vi "example_01_compress.vi"() -> ()   [LabVIEW 2015, in "lv-bin-7zip.lvlib" / "v1.lvlib"]
uses:
  v1.lvlib
  <userlib>/antonio-alexander/lv-bin/lv-bin/public/api/v1/advanced/add_data_path_multiple.vi
  advanced/compress_exe.vi
  <userlib>/antonio-alexander/lv-bin/lv-bin/public/api/v1/v1.lvlib
panel:
  in  "bin_path":path
  out "archive_path out":path
  out "error out":errorcluster
  in  "archive_path in":path
  in  "files_to_add":path
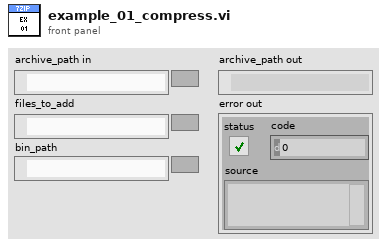
[diagram p1: front panel]
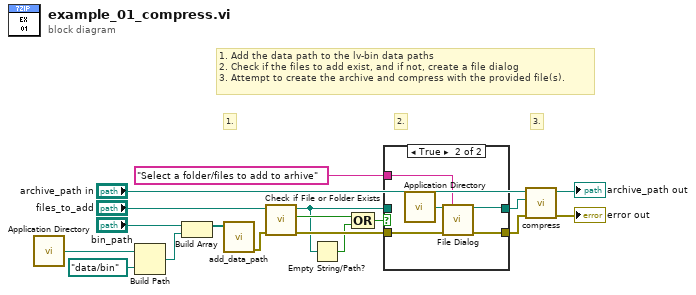
[diagram p0: block diagram]
diagram:
  # "1."
  # "1. Add the data path to the lv-bin data paths\n2. Check if the files to add exist, and if not, create a file dialog\n3. Attempt to create the archive and compress with the provided file(s)."
  # "3."
  # "2."
  n1 = call <vilib>:"Application Directory.vi"() -> ("Application Directory"=w3:path)
  n2 = Build Path(base path=w3, name or relative path=path "data/bin" ("Application Directory")) -> (appended path=w4:path)
  n3 = Build Array("bin_path", w4) -> (w6:path[])
  n4 = call-poly <userlib>:"add_data_path.vi"("path_to_add []"=w6) -> ("error out"=w5:errorcluster)  [unwired: 10 in]
  n5 = call <vilib>:"Check if File or Folder Exists.vi"("error in (no error)"=w5, "path"="files_to_add") -> ("error out"=w14:errorcluster, "file or folder exists?"=w11:bool, "dup path"=w9:path)  [unwired: 7 in]
  n6 = Empty String/Path?(string/path=w9) -> (empty?=w10:bool)
  n7 = Compound Arithmetic op=OR(w11, w10) -> (w8:bool)
  n8 = case shown="True" w8 {
    tunnel: w14 -> [w19 w25]
    tunnel: [w19 w24] -> w13
    tunnel: w9 -> [w20 _]
    tunnel: [w20 w23] -> w12
    tunnel: "Select a folder/files to add to arhive" ("prompt") -> [_ w21]
    frame False {
    }
    frame True {
      n9 = call <vilib>:"Application Directory.vi"() -> ("Application Directory"=w22:path)
      n10 = call "File Dialog"("start path"=w22, "prompt"=w21, "error in"=w25) -> ("selected path"=w23:path, "error out"=w24:errorcluster)  [unwired: 9 in, 2 out]
    }
  }
  n11 = call-poly "compress.vi"("error in (no error)"=w13, "files_to_add"=w12, "archive_path in"="archive_path in") -> ("error out"=→"error out":errorcluster, "archive_path out"=→"archive_path out":path)  [unwired: 7 in]
